vi "ke37xx Execute Scan.vi"(0 "VISA Resource Name":refnum<visa-resource-name>, 5 "Buffer Name":string, 7 "Background (False)":bool, 11 "error in (no error)":errorcluster) -> (4 "VISA Resource Name Out":refnum<visa-resource-name>, 15 "error out":errorcluster)   [LabVIEW 2009, in "Keithley 3700 Series.lvlib"]
doc: "This VI executes a scan using the existing scan list. Options are provided for executing the VI in the background and for storing the scan results in a measurement buffer."
uses:
  <instrlib>/Keithley 3706/Keithley 3700 Series.lvlib
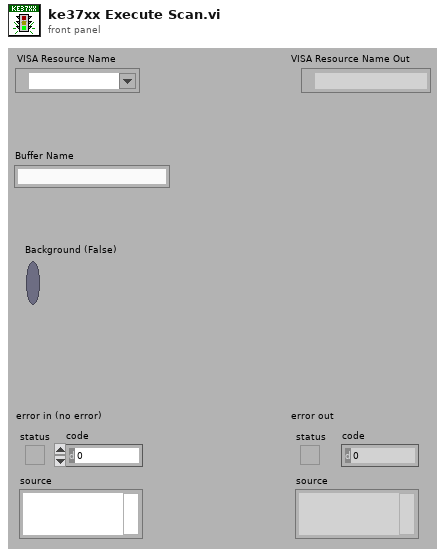
[diagram p1: front panel]
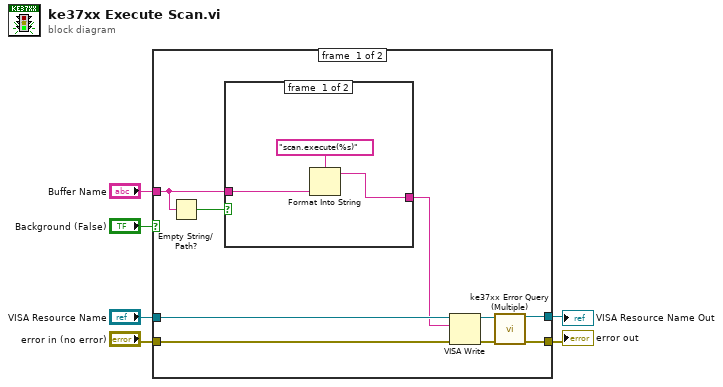
[diagram p0: block diagram]
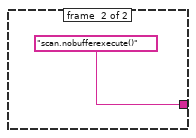
[diagram p2: hidden frame]
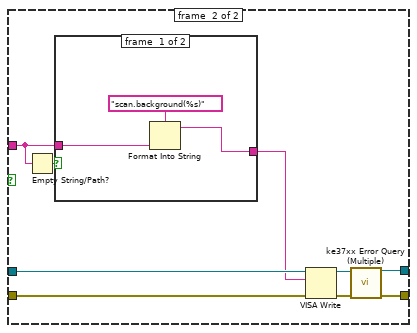
[diagram p3: hidden frame]
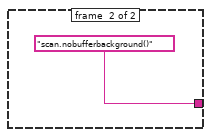
[diagram p4: hidden frame]
diagram:
  n1 = case shown="True" "Background (False)" {
    tunnel: [w15 w28] -> w6
    tunnel: [w14 w27] -> w5
    tunnel: "VISA Resource Name" -> [w13 w26]
    tunnel: "error in (no error)" -> [w12 w25]
    tunnel: "Buffer Name" -> [w7 w20]
    frame #0 {
      n2 = Empty String/Path?(string/path=w7) -> (empty?=w9:bool)
      n3 = case shown="False" w9 {
        tunnel: [w18 "scan.nobufferexecute()" ("format string")] -> w8
        tunnel: w7 -> [w17 _]
        frame #0 {
          n4 = Format Into String(format string="scan.execute(%s)", w17) -> (resulting string=w18:string)  [unwired: 2 in, 1 out]
        }
        frame #1 {
        }
      }
      n5 = VISA Write(VISA resource name=w13, write buffer=w8, error in (no error)=w12) -> (VISA resource name out=w11:refnum<visa-resource-name>, error out=w10:errorcluster)  [unwired: 1 out]
      n6 = call <instrlib>:"ke37xx Error Query (Multiple).vi"("VISA resource name"=w11, "error in (no error)"=w10) -> ("VISA resource name out"=w15:refnum<visa-resource-name>, "error out"=w14:errorcluster)  [unwired: 12 out]
    }
    frame #1 {
      n7 = Empty String/Path?(string/path=w20) -> (empty?=w22:bool)
      n8 = case shown="True" w22 {
        tunnel: [w30 "scan.nobufferbackground()" ("format string")] -> w21
        tunnel: w20 -> [w29 _]
        frame #0 {
          n9 = Format Into String(format string="scan.background(%s)", w29) -> (resulting string=w30:string)  [unwired: 2 in, 1 out]
        }
        frame #1 {
        }
      }
      n10 = VISA Write(VISA resource name=w26, write buffer=w21, error in (no error)=w25) -> (VISA resource name out=w24:refnum<visa-resource-name>, error out=w23:errorcluster)  [unwired: 1 out]
      n11 = call <instrlib>:"ke37xx Error Query (Multiple).vi"("VISA resource name"=w24, "error in (no error)"=w23) -> ("VISA resource name out"=w28:refnum<visa-resource-name>, "error out"=w27:errorcluster)  [unwired: 12 out]
    }
  }
  "VISA Resource Name Out" <- w6
  "error out" <- w5
